vi "CreateSynteticMieData.vi"(1 "Systematic Error":sgl=1.0, 4 "Uncertainty (sigma) in percentages from the mean":i32=5, 5 "Number of particle sizes of measurements":i32=5, 6 "Random Error factor":dbl, 7 "max size parameter alpha\n(alpha = 2Pi*r/lambda)":sgl=20.0 step=0.01 format="%.2f", 8 "Number of Measurements":i32=22, 9 "refractive index, imaginary":sgl step=0.01 format="%.3f", 10 "refractive index, real":sgl=1.3 step=0.01 format="%.3f") -> (0 "X Mean std error Expected extinction":T1={"Ramp Pattern"=[0.01, 5.0075, 10.005, 15.0025, 20.0], [9.193221925910608e-10, 3.2280244578654798, 2.6584865701803753, 2.2083114129269164, 2.468869368264049], [9.365225885602339e-12, 0.03861031039146786, 0.03286311037188227, 0.031522035769723275, 0.03148472361615249], [9.324156e-10, 3.261758, 2.66885, 2.2008061, 2.4853888]}, 2 "Absorption Graph":cluster{"Y":dbl[], "Y":dbl[]}[](graph), 3 "Extinction Graph":cluster{"Ramp Pattern":dbl[], dbl[]}[](graph)=[{"Ramp Pattern"=[0.01, 0.01, 0.01, 5.0075, 5.0075, 5.0075, 10.005, 10.005, 10.005, 15.0025, 15.0025, 15.0025, 20.0, 20.0, 20.0], [nan, 9.691679588472513e-10, 8.962580828507714e-10, nan, 3.509197596237534, 3.1244686343033616, nan, 2.811702731050486, 2.5256586943155415, nan, 2.314777268258088, 2.059596304910344, nan, 2.630621247591859, 2.3719335393558096]}, {"Ramp Pattern"=array[1000 elements], array[1000 elements]}, {"Ramp Pattern"=[0.01, 0.01, 0.01, 5.0075, 5.0075, 5.0075, 10.005, 10.005, 10.005, 15.0025, 15.0025, 15.0025, 20.0, 20.0, 20.0], [nan, 9.404852397449356e-10, 9.249408019530872e-10, nan, 3.357845360414006, 3.2758208701268896, nan, 2.699173109453584, 2.6381883159124433, nan, 2.214389168677243, 2.159984404491189, nan, 2.528853595827993, 2.473701191119676]}, {"Ramp Pattern"=[0.01, 5.0075, 10.005, 15.0025, 20.0], [9.32415589183222e-10, 3.2617580890655518, 2.6688499450683594, 2.200806140899658, 2.48538875579834]}])   [LabVIEW 2011]
uses:
  <vilib>/Analysis/1siggen.llb/Ramp Pattern by Samples.vi
  <vilib>/gmath/statdist.llb/Normal Random.vi
  mie2.dll
  <vilib>/Analysis/NI_AALBase.lvlib
  <vilib>/gmath/NI_Gmath.lvlib
panel:
  out "totalscatter 2":sgl=2.4853888
  out "backscatter 2":sgl=1.4156617
  out "<cos(theta)> 3":sgl=0.81333953
  out "extinction 2":sgl=2.4853888
  out "extinction":sgl=2.7353504
  in  "Number of particle sizes for expected values":i32=1000
  out "<cos(theta)> 2":sgl=0.84980327
  out "backscatter":sgl=1.1527499
  out "totalscatter":sgl=2.73535
  in  "angles (will compute\n2*angles-1 points from\n0...180 degrees)":u32=2
  # "Mie scattering demo program, August 2005, by Martin Fierz (martin@fierz.ch)\n\nThis VI demonstrates the usage of mie2.dll; a dynamic-link-library which you can call in your LabView program.\nThe demo lets you select the refractive index of a sphere, and the size parameter and computes total scattering,\ntotal extinction and angular distribution of the scattered light for p-, s- and unpolarized light.\nMie2.dll uses the Bohren-Huffman Mie code."
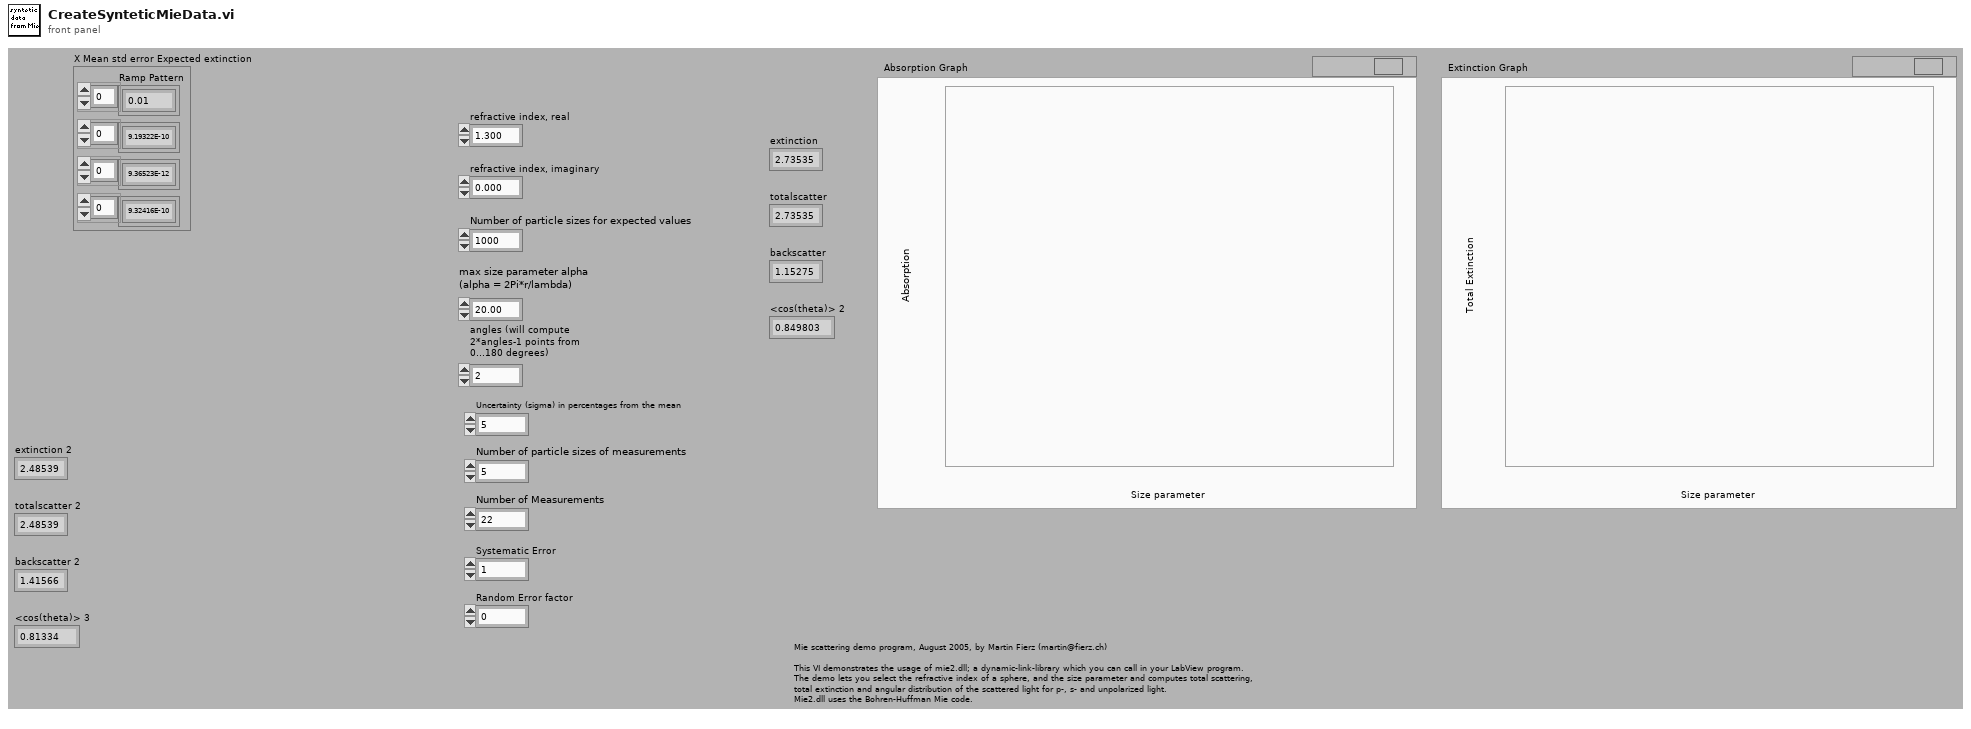
[diagram p1: front panel]
types:
  T1 = cluster{"Ramp Pattern":dbl[], dbl[], dbl[], sgl[]}
  T2 = cluster{"Ramp Pattern":dbl[], dbl[], dbl[], dbl[]}
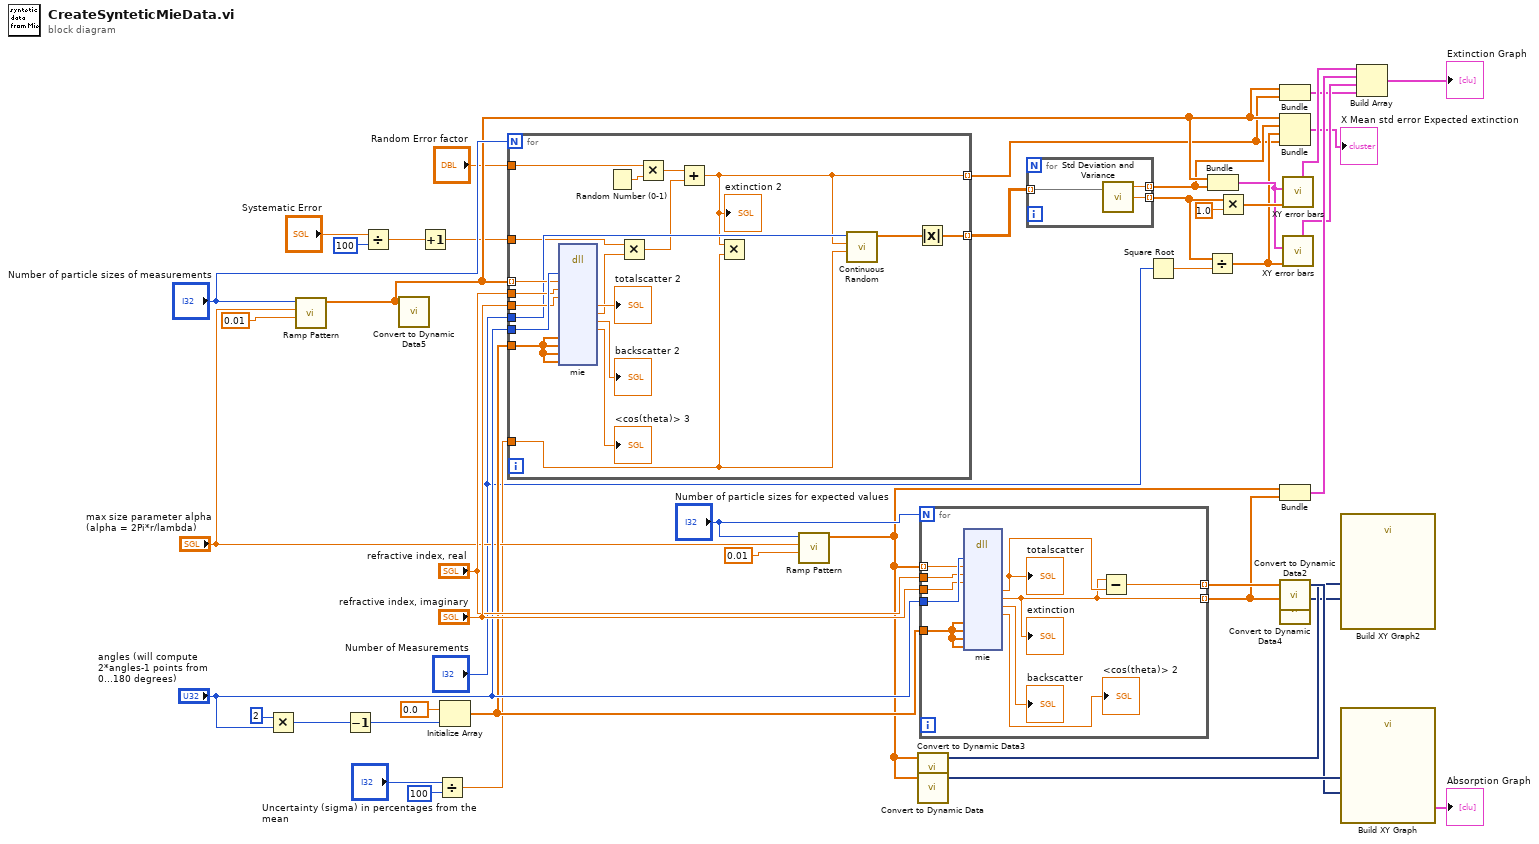
[diagram p0: block diagram]
diagram:
  n1 = Multiply(x=u32 2, y="angles (will compute\n2*angles-1 points from\n0...180 degrees)") -> (x*y=w45:u32)
  n2 = call-poly <vilib>:"Ramp Pattern.vi"("start"=0.01, "end"="max size parameter alpha\n(alpha = 2Pi*r/lambda)", "samples"="Number of particle sizes of measurements") -> ("Ramp Pattern"=w12:dbl[])  [unwired: 7 in, 1 out]
  n3 = Decrement(x=w45) -> (x-1=w43:u32)
  n4 = Divide(x="Systematic Error", y=100) -> (x/y=w4:sgl)
  n5 = call "Convert to Dynamic Data5"("Array"=w12) -> ()  [unwired: 3 in, 1 out]
  n6 = Increment(x=w4) -> (x+1=w2:sgl)
  n7 = Divide(x="Uncertainty (sigma) in percentages from the mean", y=100) -> (x/y=w26:dbl)
  n8 = Initialize Array(sgl 0.0, w43) -> (w31:sgl[])
  n9 = for {
    N: "Number of particle sizes of measurements" -> [_]
    tunnel: w31 -> [w63]
    tunnel: "angles (will compute\n2*angles-1 points from\n0...180 degrees)" -> [w62]
    tunnel: "refractive index, real" -> [w61]
    tunnel: "refractive index, imaginary" -> [w60]
    tunnel: w12 -> [w59] mode=indexing
    tunnel: w26 -> [w49]
    tunnel: [w47] -> w25 mode=indexing
    tunnel: "Number of Measurements" -> [w57]
    tunnel: [w50] -> w6 mode=indexing
    tunnel: w2 -> [w52]
    tunnel: "Random Error factor" -> [w53]
    n10 = dll-call lib="Y:/Lior Segev/Lior Segev Projects/BAES data analysis/mie2.dll" fn="mie"("angles"=w62, "x"=w59, "r"=w61, "i"=w60, "spol_real"=w63, "spol_imaginary"=w63, "ppol_real"=w63, "ppol_imaginary"=w63) -> ("totalscatter"=→"totalscatter 2":sgl, "extinction"=w56:sgl, "backscatter"=→"backscatter 2":sgl, "<cos(theta)>"=→"<cos(theta)> 3":sgl)  [unwired: 16 in, 2 out]
    n11 = Random Number (0-1)() -> (number: 0 to 1=w55:dbl)
    n12 = Multiply(x=w52, y=w56) -> (x*y=w51:sgl)
    n13 = Multiply(x=w53, y=w55) -> (x*y=w54:dbl)
    n14 = Add(x=w54, y=w51) -> (x+y=w50:dbl)
    "extinction 2" <- w50
    n15 = Multiply(x=w50, y=w49) -> ()  [unwired: 1 out]
    n16 = call-poly <vilib>:"Continuous Random.vi"("std"=w49, "mean"=w50, "samples"=w57) -> ("normal random data"=w48:dbl[])  [unwired: 7 in, 1 out]
    n17 = Absolute Value(x=w48) -> (abs(x)=w47:dbl[])
  }
  n18 = call-poly <vilib>:"Ramp Pattern.vi"("start"=0.01, "end"="max size parameter alpha\n(alpha = 2Pi*r/lambda)", "samples"="Number of particle sizes for expected values") -> ("Ramp Pattern"=w22:dbl[])  [unwired: 7 in, 1 out]
  n19 = call "Convert to Dynamic Data3"("Array"=w22) -> ("Dynamic Data Type"=w36:dynamicdata)  [unwired: 3 in]
  n20 = call "Convert to Dynamic Data"("Array"=w22) -> ("Dynamic Data Type"=w41:dynamicdata)  [unwired: 3 in]
  n21 = for {
    N: "Number of particle sizes for expected values" -> [_]
    tunnel: w31 -> [w73]
    tunnel: "angles (will compute\n2*angles-1 points from\n0...180 degrees)" -> [w72]
    tunnel: "refractive index, real" -> [w71]
    tunnel: "refractive index, imaginary" -> [w70]
    tunnel: [w67] -> w40 mode=indexing
    tunnel: w22 -> [w69] mode=indexing
    tunnel: [w66] -> w8 mode=indexing
    n22 = dll-call lib="Y:/Lior Segev/Lior Segev Projects/BAES data analysis/mie2.dll" fn="mie"("angles"=w72, "x"=w69, "r"=w71, "i"=w70, "spol_real"=w73, "spol_imaginary"=w73, "ppol_real"=w73, "ppol_imaginary"=w73) -> ("totalscatter"=w68:sgl, "extinction"=w66:sgl, "backscatter"=→"backscatter":sgl, "<cos(theta)>"=→"<cos(theta)> 2":sgl)  [unwired: 16 in, 2 out]
    "totalscatter" <- w68
    "extinction" <- w66
    n23 = Subtract(x=w66, y=w68) -> (x-y=w67:sgl)
  }
  n24 = for {
    tunnel: w25 -> [w78] mode=indexing
    tunnel: [w77] -> w11 mode=indexing
    tunnel: [w76] -> w17 mode=indexing
    n25 = call <vilib>:"Std Deviation and Variance.vi"("X"=w78) -> ("mean"=w77:dbl, "standard deviation"=w76:dbl)  [unwired: 1 in, 1 out]
  }
  n26 = Square Root(x="Number of Measurements") -> (sqrt(x)=w24:dbl)
  n27 = Divide(x=w17, y=w24) -> (x/y=w9:dbl[])
  n28 = Bundle("Ramp Pattern"=w12, w11) -> (w15:cluster{"Ramp Pattern":dbl[], dbl[]})  [unwired: 1 in]
  n29 = Multiply(x=w17, y=1.0) -> (x*y=w16:dbl[])
  n30 = Bundle("Ramp Pattern"=w12, w6) -> (w13:cluster{"Ramp Pattern":dbl[], dbl[]})  [unwired: 1 in]
  n31 = Bundle("Ramp Pattern"=w12, w11, w9, w6) -> (→"X Mean std error Expected extinction":T2)  [unwired: 1 in]
  n32 = Bundle("Ramp Pattern"=w22, w8) -> (w20:cluster{"Ramp Pattern":dbl[], sgl[]})  [unwired: 1 in]
  n33 = call "Convert to Dynamic Data2"("Array"=w40) -> ("Dynamic Data Type"=w39:dynamicdata)  [unwired: 3 in]
  n34 = call "Convert to Dynamic Data4"("Array"=w8) -> ("Dynamic Data Type"=w35:dynamicdata)  [unwired: 3 in]
  n35 = call "XY error bars.vi"("XY plot"=w15, "Yerror"=w16) -> ("Y error bars"=w21:cluster{dbl[], dbl[]})  [unwired: 6 in, 2 out]
  n36 = call "XY error bars.vi"("XY plot"=w15, "Yerror"=w9) -> ("Y error bars"=w14:cluster{dbl[], dbl[]})  [unwired: 6 in, 2 out]
  n37 = call "Build XY Graph2"("Y Input"=w35, "X Input"=w36) -> ()  [unwired: 3 in, 7 out]
  n38 = call "Build XY Graph"("Y Input"=w39, "X Input"=w41) -> ("XY Graph"=→"Absorption Graph":cluster{"Y":dbl[], "Y":dbl[]}[])  [unwired: 3 in, 6 out]
  n39 = Build Array(w21, w20, w14, w13) -> (→"Extinction Graph":cluster{"Ramp Pattern":dbl[], dbl[]}[])
